vi "Initialise Data Bus Task.vi"(8 "error in":errorcluster) -> (0 "error out":errorcluster, 3 "Data Bus":refnum<k21> caption="task out")   [LabVIEW 2021, in "IO.lvclass"]
uses:
  IO.lvclass
  <vilib>/DAQmx/create/channels.llb/DAQmx Create Channel (DO-Digital Output).vi
  IO.lvclass/IO.ctl
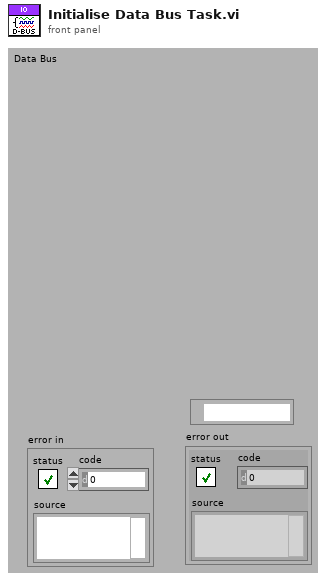
[diagram p1: front panel]
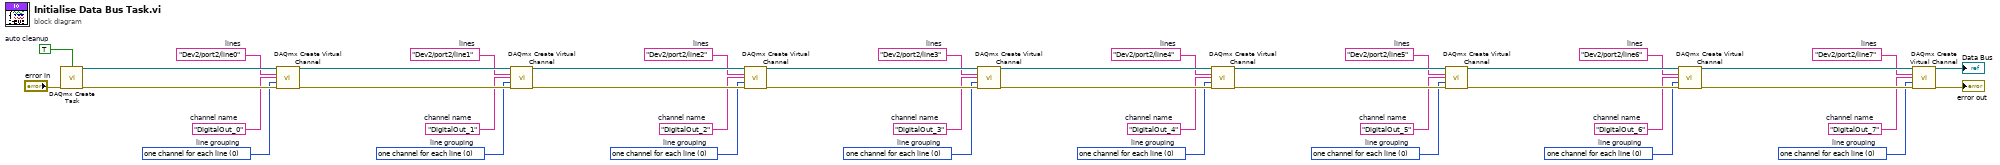
[diagram p0: block diagram]
diagram:
  w4 = 0 items=["one channel for each line", "one channel for all lines"]  # line grouping
  w3 = "DigitalOut_7"  # channel name
  w5 = "Dev2/port2/line7"  # lines
  w9 = 0 items=["one channel for each line", "one channel for all lines"]  # line grouping
  w8 = "DigitalOut_6"  # channel name
  w10 = "Dev2/port2/line6"  # lines
  w14 = 0 items=["one channel for each line", "one channel for all lines"]  # line grouping
  w13 = "DigitalOut_5"  # channel name
  w15 = "Dev2/port2/line5"  # lines
  w19 = 0 items=["one channel for each line", "one channel for all lines"]  # line grouping
  w18 = "DigitalOut_4"  # channel name
  w20 = "Dev2/port2/line4"  # lines
  w24 = 0 items=["one channel for each line", "one channel for all lines"]  # line grouping
  w23 = "DigitalOut_3"  # channel name
  w25 = "Dev2/port2/line3"  # lines
  w29 = 0 items=["one channel for each line", "one channel for all lines"]  # line grouping
  w28 = "DigitalOut_2"  # channel name
  w30 = "Dev2/port2/line2"  # lines
  w34 = 0 items=["one channel for each line", "one channel for all lines"]  # line grouping
  w33 = "DigitalOut_1"  # channel name
  w35 = "Dev2/port2/line1"  # lines
  w39 = 0 items=["one channel for each line", "one channel for all lines"]  # line grouping
  w38 = "DigitalOut_0"  # channel name
  w40 = "Dev2/port2/line0"  # lines
  w42 = TRUE  # auto cleanup
  n1 = call <vilib>:"DAQmx Create Task.vi"("auto cleanup"=w42, "error in"="error in") -> ("task out"=w41:refnum<k21>, "error out"=w43:errorcluster)  [unwired: 12 in]
  n2 = call-poly <vilib>:"DAQmx Create Virtual Channel.vi"("task in"=w41, "lines"=w40, "name to assign"=w38, "line grouping"=w39, "error in"=w43) -> ("task out"=w36:refnum<k21>, "error out"=w37:errorcluster)  [unwired: 9 in]
  n3 = call-poly <vilib>:"DAQmx Create Virtual Channel.vi"("task in"=w36, "lines"=w35, "name to assign"=w33, "line grouping"=w34, "error in"=w37) -> ("task out"=w31:refnum<k21>, "error out"=w32:errorcluster)  [unwired: 9 in]
  n4 = call-poly <vilib>:"DAQmx Create Virtual Channel.vi"("task in"=w31, "lines"=w30, "name to assign"=w28, "line grouping"=w29, "error in"=w32) -> ("task out"=w26:refnum<k21>, "error out"=w27:errorcluster)  [unwired: 9 in]
  n5 = call-poly <vilib>:"DAQmx Create Virtual Channel.vi"("task in"=w26, "lines"=w25, "name to assign"=w23, "line grouping"=w24, "error in"=w27) -> ("task out"=w21:refnum<k21>, "error out"=w22:errorcluster)  [unwired: 9 in]
  n6 = call-poly <vilib>:"DAQmx Create Virtual Channel.vi"("task in"=w21, "lines"=w20, "name to assign"=w18, "line grouping"=w19, "error in"=w22) -> ("task out"=w16:refnum<k21>, "error out"=w17:errorcluster)  [unwired: 9 in]
  n7 = call-poly <vilib>:"DAQmx Create Virtual Channel.vi"("task in"=w16, "lines"=w15, "name to assign"=w13, "line grouping"=w14, "error in"=w17) -> ("task out"=w11:refnum<k21>, "error out"=w12:errorcluster)  [unwired: 9 in]
  n8 = call-poly <vilib>:"DAQmx Create Virtual Channel.vi"("task in"=w11, "lines"=w10, "name to assign"=w8, "line grouping"=w9, "error in"=w12) -> ("task out"=w6:refnum<k21>, "error out"=w7:errorcluster)  [unwired: 9 in]
  n9 = call-poly <vilib>:"DAQmx Create Virtual Channel.vi"("task in"=w6, "lines"=w5, "name to assign"=w3, "line grouping"=w4, "error in"=w7) -> ("task out"=→"Data Bus":refnum<k21>, "error out"=→"error out":errorcluster)  [unwired: 9 in]
